vi "Header.vi"(3 "GeneralResult":string, 5 "P/N UUT":string, 9 "Driver S/N":string, 11 "error in":errorcluster, 13 "Oper.":string, 14 "Tester Software Ver":string) -> (6 "Array":string[][](array[string]), 15 "error out":errorcluster)   [LabVIEW 2017]
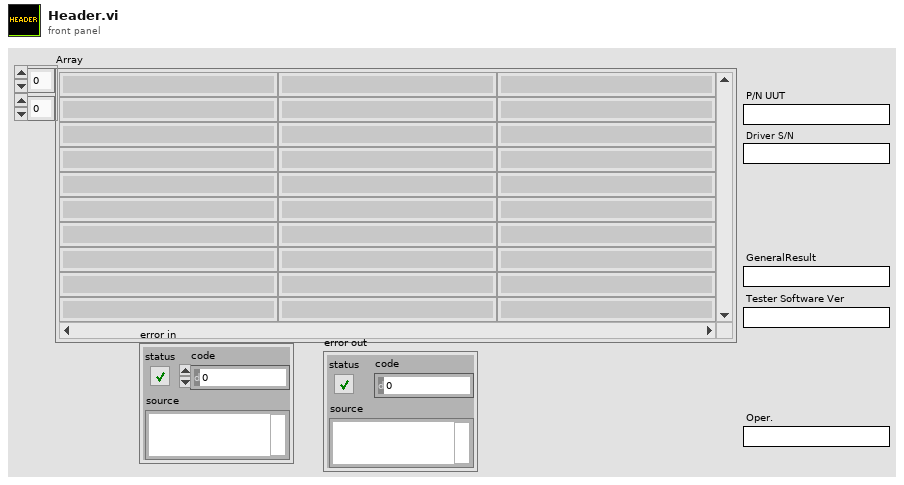
[diagram p1: front panel]
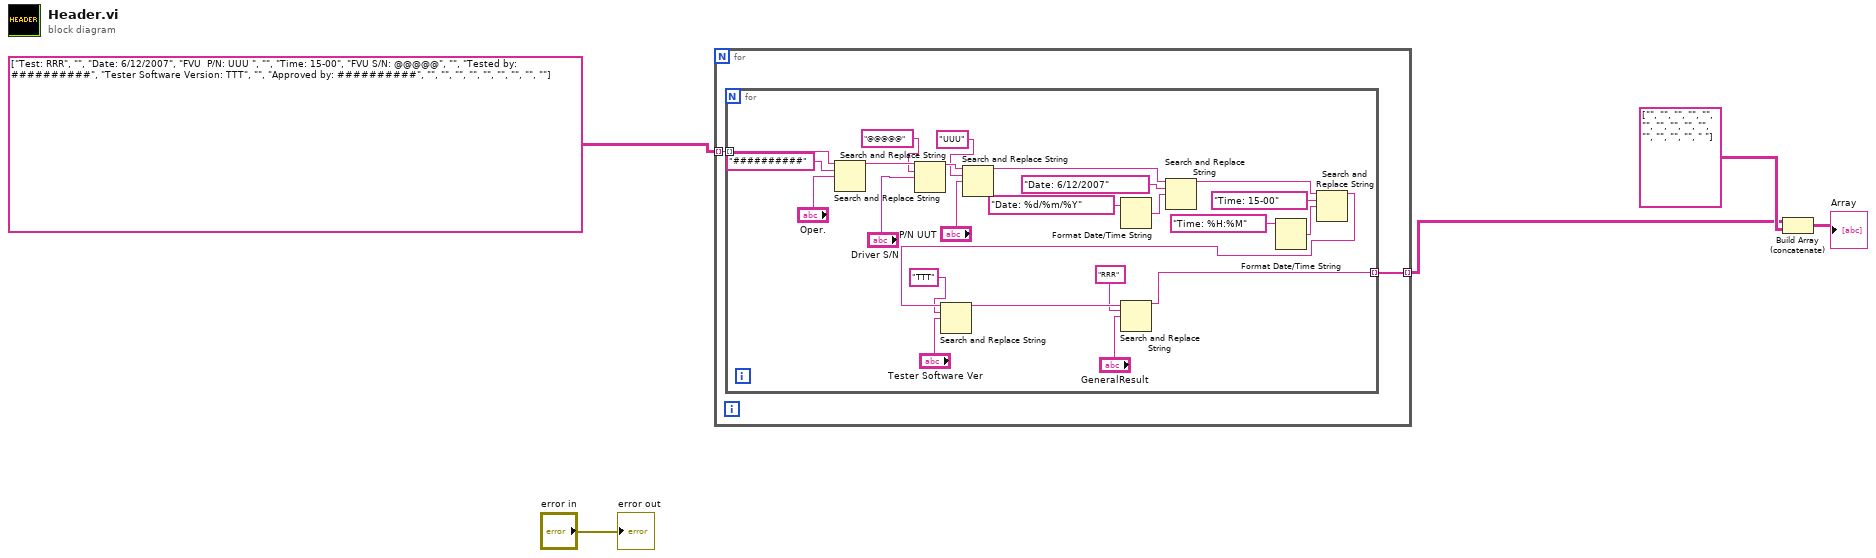
[diagram p0: block diagram]
diagram:
  n1 = for {
    tunnel: string[][] [["Test: RRR", "", "Date: 6/12/2007"], ["FVU  P/N: UUU ", "", "Time: 15-00"], ["FVU S/N: @@@@@", "", "Tested by: ##########"], ["Tester Software Version: TTT", "", "Approved by: ##########"], ["", "", ""], ["", "", ""], ["", "", ""]] -> [w7] mode=indexing
    tunnel: [w6] -> w2 mode=indexing
    n2 = for {
      tunnel: w7 -> [w9] mode=indexing
      tunnel: [w8] -> w6 mode=indexing
      n3 = Search and Replace String(input string=w9, search string="##########" ("source"), replace string="Oper.") -> (result string=w20:string)  [unwired: 5 in, 3 out]
      n4 = Search and Replace String(input string=w20, search string="@@@@@" ("source"), replace string="Driver S/N") -> (result string=w22:string)  [unwired: 5 in, 3 out]
      n5 = Search and Replace String(input string=w22, search string="UUU" ("source"), replace string="P/N UUT") -> (result string=w21:string)  [unwired: 5 in, 3 out]
      n6 = Format Date/Time String(time format string (%c)="Date: %d/%m/%Y") -> (date/time string=w19:string)  [unwired: 2 in]
      n7 = Search and Replace String(input string=w21, search string="Date: 6/12/2007" ("time format string (%c)"), replace string=w19) -> (result string=w28:string)  [unwired: 5 in, 3 out]
      n8 = Format Date/Time String(time format string (%c)="Time: %H:%M") -> (date/time string=w30:string)  [unwired: 2 in]
      n9 = Search and Replace String(input string=w28, search string="Time: 15-00", replace string=w30) -> (result string=w29:string)  [unwired: 5 in, 3 out]
      n10 = Search and Replace String(input string=w29, search string="TTT", replace string="Tester Software Ver") -> (result string=w27:string)  [unwired: 5 in, 3 out]
      n11 = Search and Replace String(input string=w27, search string="RRR", replace string="GeneralResult") -> (result string=w8:string)  [unwired: 5 in, 3 out]
    }
  }
  n12 = Build Array (concatenate)(w2, string[][] [["", "", ""], ["", "", ""], ["", "", ""], ["", "", ""], ["", "", " "]]) -> (→"Array":string[][])
  "error out" <- "error in"
